vi "CRYNoise White Pink.vi"(0 "Fs":dbl=1.0 format="%.2f", 1 "Setting Infor":T2 {"dB ref" format="%#_6p"}, 2 "EQ Curve":T1={"Name"="", "Curve"=[], "X data"=1, "Y data"=1, "Z data"=1, "X axis"=0, "Y axis"=1, "Z axis"=1, "X unit"="Hz", "Y unit"="", "Z unit"="deg.", "X dB ref"=1.0, "Y dB ref"=1.0, "Z dB ref"=1.0, "single val"=FALSE, "protected"=FALSE, "display X"=TRUE, "display Y"=TRUE, "display Z"=TRUE, "Test Info"="", "Step No."=0, "Plot Settings"={"Color"=0, "Interpolation"=0, "Point Style"=0, "Line Style"=0, "Point Color"=0, "Line Width"=0, "Bar Plot Style"=0, "Fill To"=0}, "AutoProtect"=FALSE} {"Z data" items=["dB", "Lin"]; "X data" items=["dB", "Lin"]; "Y data" items=["dB", "Lin"]; "Z dB ref" format="%.1f"; "Z axis" items=["Log", "Lin"]; "X dB ref" format="%.1f"; "X axis" items=["Log", "Lin"]; "Y axis" items=["Log", "Lin"]; "Y dB ref" format="%.1f"; "Curve"."z" format="%.2f"; "Curve"."y" format="%.2f"; "Curve"."x" format="%.2f"}, 3 "Output Flag":cluster{bool, bool, "ApplyEQ":bool}, 5 "Min Frequency":dbl=1.0 format="%.2f", 7 "Max Frequency":dbl=1.0 format="%.2f", 9 "Time(s)":dbl=1.0 format="%.2f", 11 "error in (no error)":errorcluster, 12 "Amplitude":dbl=1.0 format="%.2p", 13 "Noise type":u16(ring)=1 items=["White Noise", "Pink Noise"]) -> (4 "Noise":sgl[](array[numeric]), 6 "sample size":u32, 8 "rms value":dbl format="%.2p", 15 "error out":errorcluster)   [LabVIEW 2013]
uses:
  Typedef Control/CRYData Cluster.ctl
  <vilib>/Analysis/5stat.llb/RMS (DBL).vi
  <vilib>/Analysis/NI_AALPro.lvlib
  <vilib>/Analysis/NI_AALBase.lvlib
panel:
  out "Waveform Graph":dbl[](graph)
  out "Crest Factor":sgl
  out "Max Out":sgl format="%#_6p"
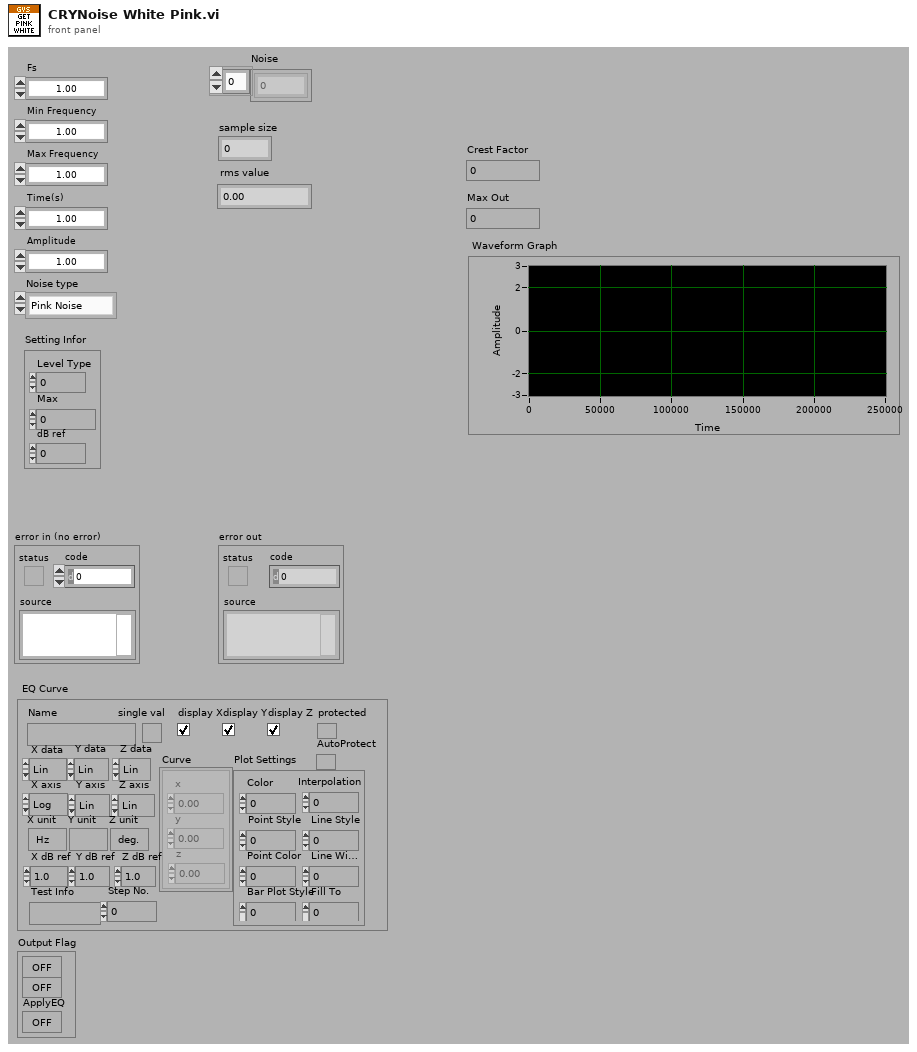
[diagram p1: front panel]
types:
  T1 = typedef "CRYData Cluster.ctl" = cluster{"Name":string, "Curve":cluster{"x":dbl, "y":dbl, "z":dbl}[], "X data":u16, "Y data":u16, "Z data":u16, "X axis":u16, "Y axis":u16, "Z axis":u16, "X unit":string, "Y unit":string, "Z unit":string, "X dB ref":dbl, "Y dB ref":dbl, "Z dB ref":dbl, "single val":bool, "protected":bool, "display X":bool, "display Y":bool, "display Z":bool, "Test Info":string, "Step No.":i32, "Plot Settings":cluster{"Color":u32, "Interpolation":u8, "Point Style":u8, "Line Style":u8, "Point Color":u32, "Line Width":u8, "Bar Plot Style":u8, "Fill To":i16}, "AutoProtect":bool}
  T2 = cluster{"Level Type":u16, "Max":dbl, "dB ref":dbl}
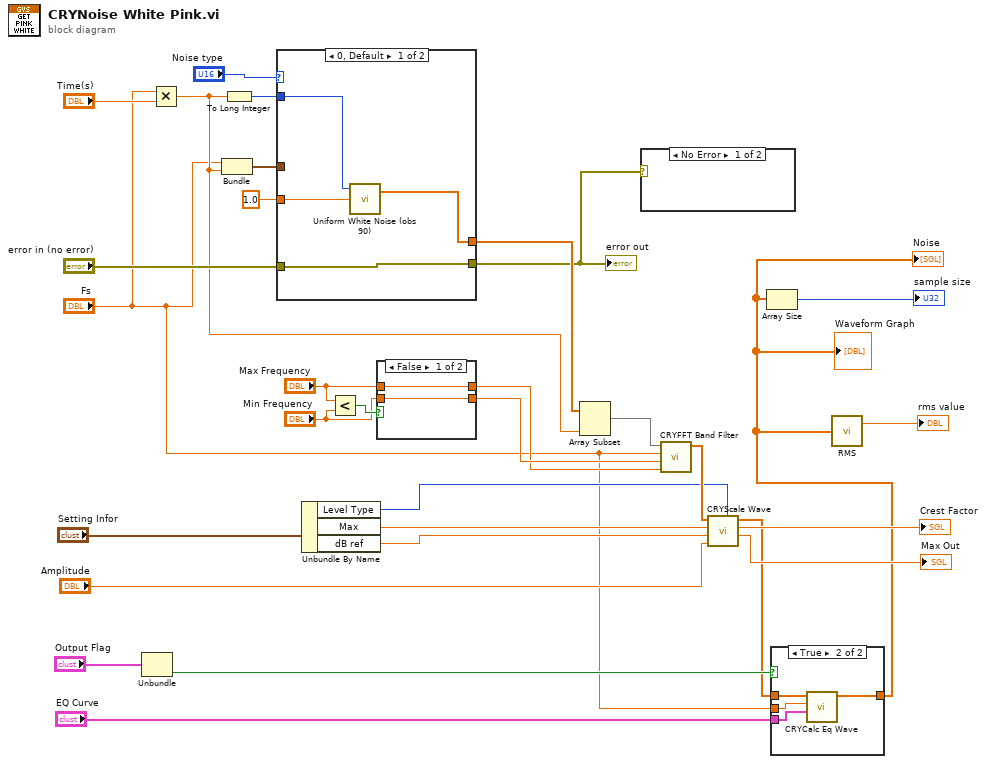
[diagram p0: block diagram]
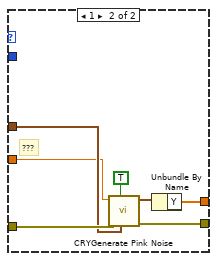
[diagram p5: hidden frame]
diagram:
  n1 = Unbundle("Output Flag") -> ("ApplyEQ"=w4:bool)  [unwired: 2 out]
  n2 = Multiply(x="Fs", y="Time(s)") -> (x*y=w21:dbl)
  n3 = Bundle("Fs"="Fs", w21) -> (w29:cluster{"Fs":dbl, dbl})  [unwired: 1 in]
  n4 = To Long Integer(number=w21) -> (32bit integer=w27:i32)
  n5 = case shown="0, Default" "Noise type" {
    tunnel: 1.0 ("Amplitude") -> [w32 w36]
    tunnel: "error in (no error)" -> [w33 w40]
    tunnel: [w33 w39] -> w16
    tunnel: w29 -> [_ w37]
    tunnel: [w35 w42] -> w20
    tunnel: w27 -> [w34 _]
    frame 0, Default {
      n6 = call <vilib>:"Uniform White Noise (obs 90).vi"("amplitude"=w32, "samples"=w34) -> ("uniform white noise"=w35:dbl[])  [unwired: 1 in, 1 out]
    }
    frame 1 {
      # "???"
      n7 = call "CRYGenerate Pink Noise.vi"("sampling info"=w37, "reset signal (F)"=TRUE, "error in (no error)"=w40, "amplitude"=w36) -> ("error out"=w39:errorcluster, "pink noise signal"=w38:waveform(dbl))  [unwired: 1 in, 5 out]
      n8 = Unbundle By Name(w38) -> ("Y"=w42:dbl[])
    }
  }
  "error out" <- w16
  n9 = Unbundle By Name("Setting Infor") -> ("Level Type"=w10:u16, "Max"=w9:dbl, "dB ref"=w8:dbl)
  n10 = Less?(x="Max Frequency", y="Min Frequency") -> (x < y?=w26:bool)
  n11 = case shown="False" w26 {
    tunnel: "Max Frequency" -> [w43 w46]
    tunnel: "Min Frequency" -> [w44 w45]
    tunnel: [w43 w45] -> w18
    tunnel: [w44 w46] -> w19
    frame False {
    }
    frame True {
    }
  }
  n12 = Array Subset(array=w20, length=w21) -> (w17:dbl[])  [unwired: 1 in]
  n13 = case shown="No Error" w16 {
    frame No Error {
    }
    frame Error {
    }
  }
  n14 = call "CRYFFT Band Filter.vi"("High Freq"=w18, "Low Freq"=w19, "Fs"="Fs", "Signal In"=w17) -> ("Signal out"=w14:dbl[])  [unwired: 7 in]
  n15 = call "CRYScale Wave.vi"("Level Type"=w10, "Level"="Amplitude", "dB ref"=w8, "Max"=w9, "Wave"=w14) -> ("Max Out"=→"Max Out":sgl, "Crest Factor"=→"Crest Factor":sgl, "Scaled Wave"=w3:sgl[])  [unwired: 4 in]
  n16 = case shown="True" w4 {
    tunnel: "EQ Curve" -> [_ w51]
    tunnel: "Fs" -> [_ w50]
    tunnel: w3 -> [w47 w49]
    tunnel: [w47 w48] -> w2
    frame False {
    }
    frame True {
      n17 = call "CRYCalc Eq Wave.vi"("EQ Curve"=w51, "Fs"=w50, "Wave In"=w49) -> ("Wave Out"=w48:dbl[])  [unwired: 7 in, 1 out]
    }
  }
  "Noise" <- w2
  "Waveform Graph" <- w2
  n18 = Array Size(array=w2) -> (size(s)=→"sample size":i32)
  n19 = call-poly <vilib>:"RMS.vi"("X"=w2) -> ("rms value"=→"rms value":dbl)  [unwired: 1 out]
